vi "Read Write Config.vi"(8 "error in (no error)":errorcluster, 9 "Data in":variant, 10 "Command":string, 11 "config ref in":T1) -> (0 "error out":errorcluster, 1 "Data out":variant, 3 "config ref out":T1)   [LabVIEW 2018, in "Configuration.lvlib"]
uses:
  Configuration.lvlib
  <vilib>/Utility/config.llb/Config Data RefNum.ctl
  <vilib>/Utility/config.llb/Read Key (String).vi
  <vilib>/Utility/config.llb/Write Key (String).vi
  <vilib>/regexp/Match Regular Expression.xnode
  <vilib>/Utility/config.llb/NI_LVConfig.lvlib
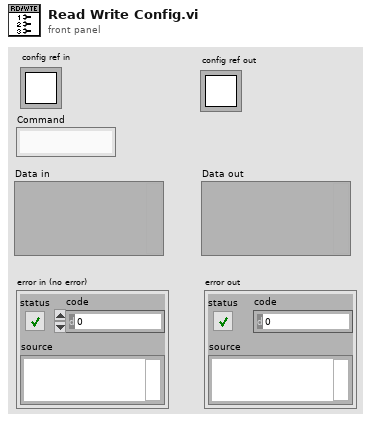
[diagram p1: front panel]
types:
  T1 = typedef "NI_LVConfig.lvlib/Config Data RefNum.ctl" = refnum<k1>
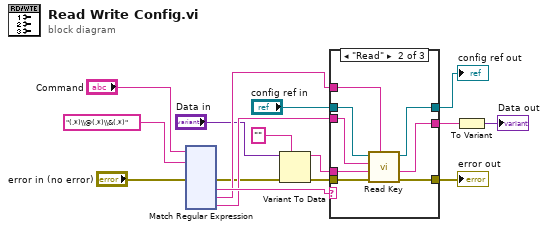
[diagram p0: block diagram]
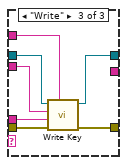
[diagram p3: hidden frame]
diagram:
  n1 = xnode "Match Regular Expression"("input string"="Command", "regular expression"="(.*)\\@(.*)\\&(.*)", "error in"="error in (no error)") -> ("error out"=w2:errorcluster, "submatch 1"=w16:string, "submatch 2"=w13:string, "submatch 3"=w12:string)  [unwired: 3 in, 4 out]
  n2 = Variant To Data(error in=w2, type="", Variant="Data in") -> (data=w9:string, error out=w3:errorcluster)
  n3 = case shown="\"Read\"" w16 {
    tunnel: w13 -> [_ w25 w32]
    tunnel: w12 -> [_ w24 w31]
    tunnel: w9 -> [_ w23 w30]
    tunnel: w3 -> [w17 w22 w29]
    tunnel: [w17 w21 w28] -> w8
    tunnel: "config ref in" -> [_ w20 w27]
    tunnel: [_ w19 w26] -> w6
    tunnel: [_ w18 _] -> w5
    frame Default {
    }
    frame "Read" {
      n4 = call-poly <vilib>:"Read Key.vi"("section"=w25, "error in (no error)"=w22, "default value"=w23, "key"=w24, "refnum"=w20) -> ("error out"=w21:errorcluster, "value"=w18:string, "refnum out"=w19:T1)  [unwired: 3 in, 1 out]
    }
    frame "Write" {
      n5 = call-poly <vilib>:"Write Key.vi"("section"=w32, "error in (no error)"=w29, "value"=w30, "key"=w31, "refnum"=w27) -> ("error out"=w28:errorcluster, "refnum out"=w26:T1)  [unwired: 4 in, 1 out]
    }
  }
  "error out" <- w8
  "config ref out" <- w6
  n6 = To Variant(anything=w5) -> (Variant=→"Data out":variant)
